vi "RunDelay2.vi"() -> ()   [LabVIEW 2009]
uses:
  BME Beispiele/BME DLL/DelayGenerator.dll
panel:
  out "error out":errorcluster
  in  "DEACTIVATE":bool
  out "output param 21":i32
  out "output param 13":i32
  out "output param 18":i32
  out "output param 7":u32
  out "output param 6":u32
  out "output param 17":i32
  out "output param 12":i32
  out "output param 11":i32
  in  "Internal Trigger":bool=TRUE
  in  "Trigger Period":dbl=10000.0
  out "output param 9":i32
  out "output param 8":i32
  in  "stop":bool
  in  "T(S) Delay":dbl
  in  "T(S) Reset":dbl
  in  "T(S) Active":bool=TRUE
  in  "A(S) Delay":dbl
  in  "A(S) Reset":dbl
  in  "A(S) Acitve":bool=TRUE
  in  "B(S) Delay":dbl=1000.0
  in  "B(S) Reset":dbl=4000.0
  in  "B(S) Acitve":bool=TRUE
  out "output param 14":u32
  out "output param 15":u32
  out "output param 16":u32
  out "output param 10":i32
  in  "T0 Active":bool=TRUE
  in  "T0 Delay":dbl
  in  "A  Delay":dbl
  in  "A  Active":bool=TRUE
  in  "B  Delay":dbl=1000.0
  in  "B  Active":bool=TRUE
  in  "Gate AB":bool=TRUE
  in  "Apply":bool
  out "output param 20":u32
  out "output param 19":u32
  out "output param 4":i32
  out "output param 5":i32
  out "output param 2":i32
  out "DG_ProductM":i32
  out "SlotNumberM":i32
  out "IsMaster?m":i32
  out "output param 3":i32
  out "DG_ProductS":i32
  out "SlotNumberS":i32
  out "IsMaster?s":i32
  out "DG_NumberM":i32
  out "DG_NumberS":i32
  out "output param 1":i32
  out "NumberOfCards Detected":i32
  out "p_Error 2":i32
  # "Info-Master"
  # "Info-Slave1"
  # "All error indicators are hidden.\nIn order to see a return value \nof some function, make the \nindicator visible (show indicator)"
  # "ALL TIME VALUES IN msek !"
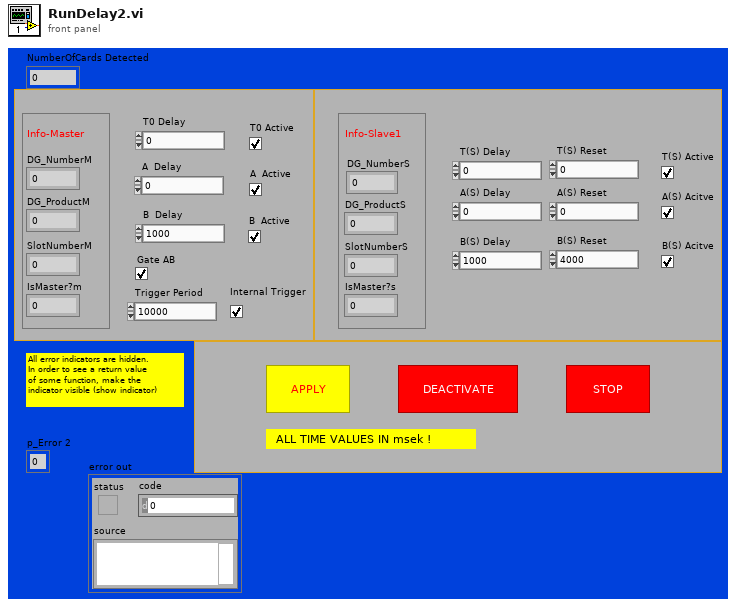
[diagram p1: front panel]
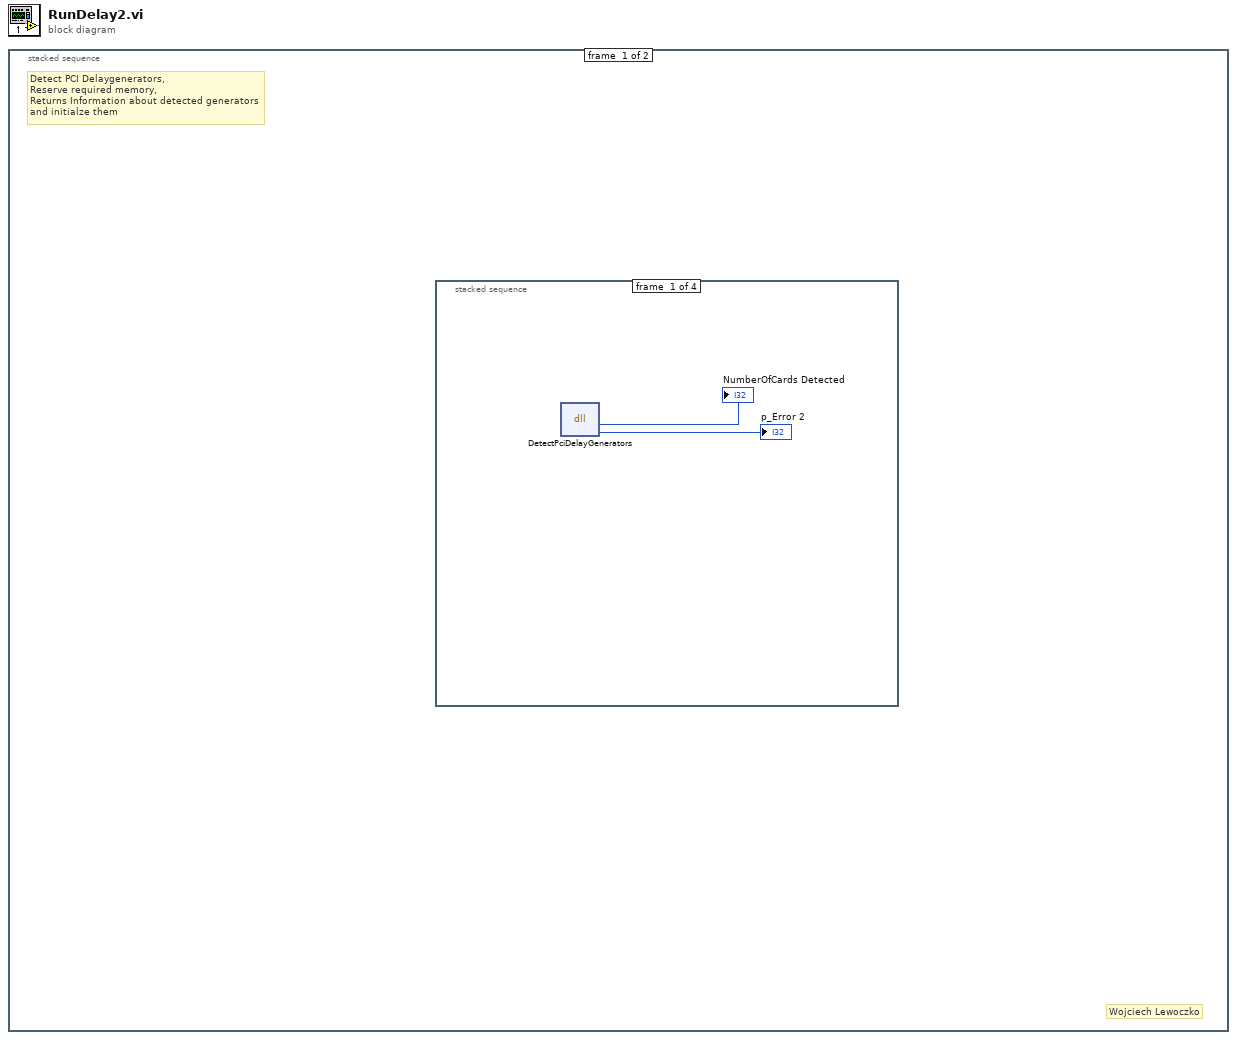
[diagram p0: block diagram]
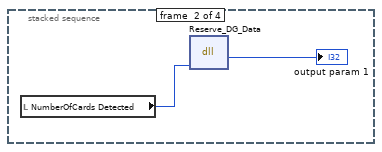
[diagram p2: hidden frame]
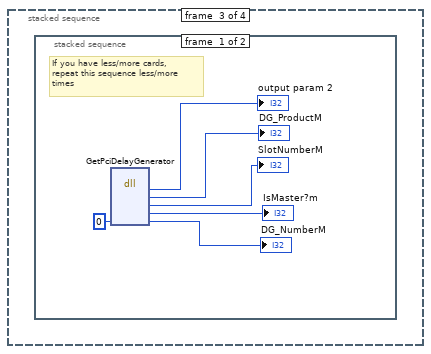
[diagram p3: hidden frame]
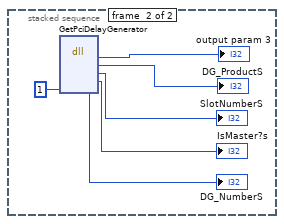
[diagram p4: hidden frame]
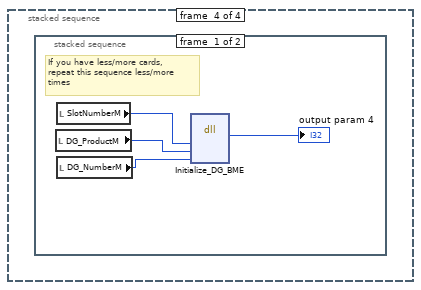
[diagram p5: hidden frame]
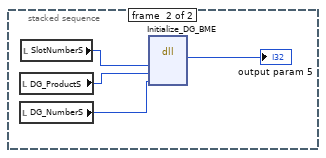
[diagram p6: hidden frame]
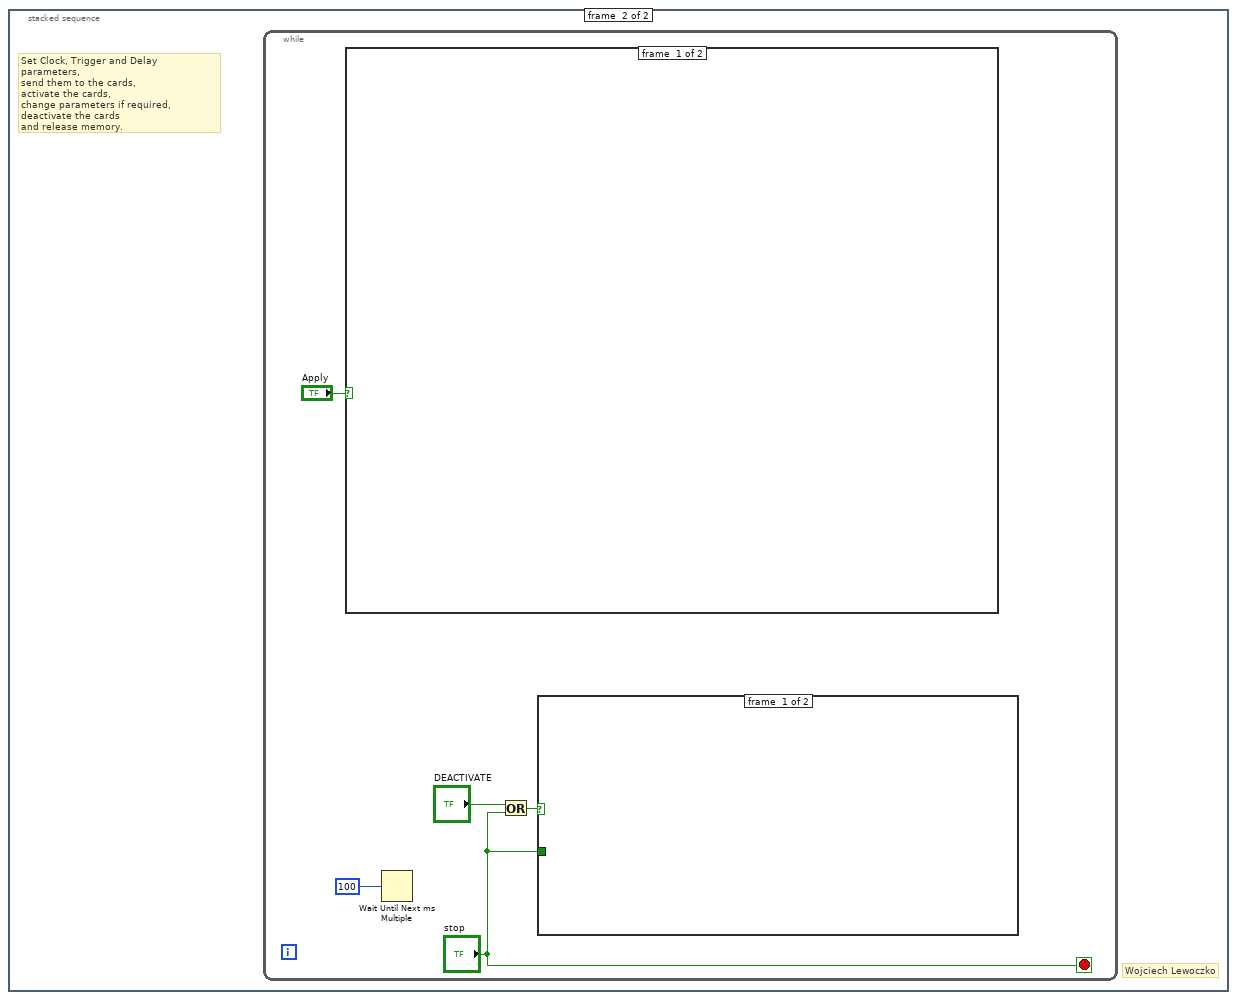
[diagram p7: hidden frame]
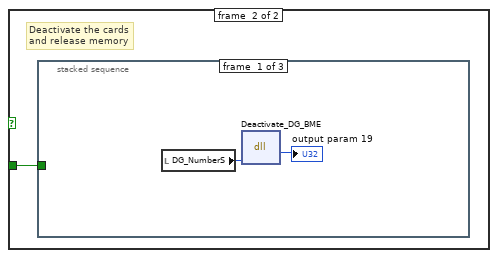
[diagram p8: hidden frame]
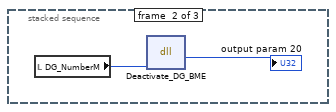
[diagram p9: hidden frame]
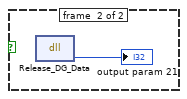
[diagram p11: hidden frame]
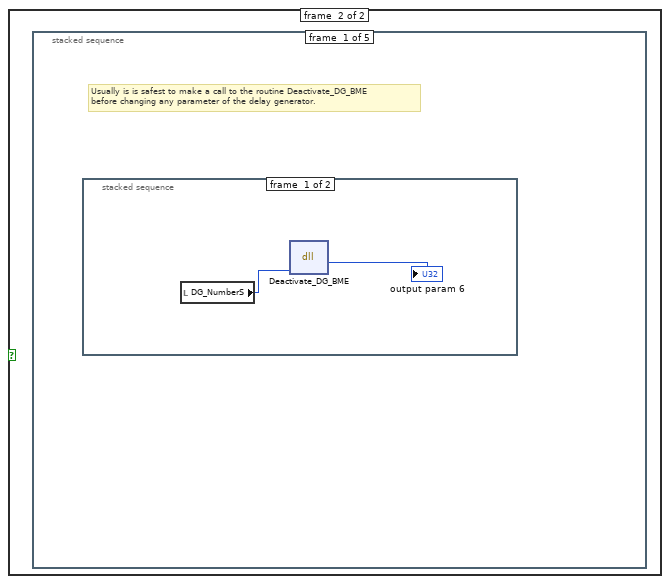
[diagram p12: hidden frame]
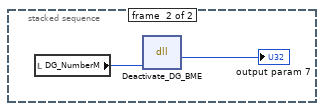
[diagram p13: hidden frame]
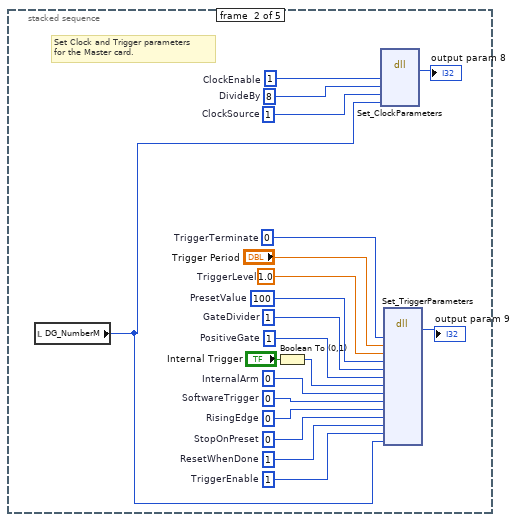
[diagram p14: hidden frame]
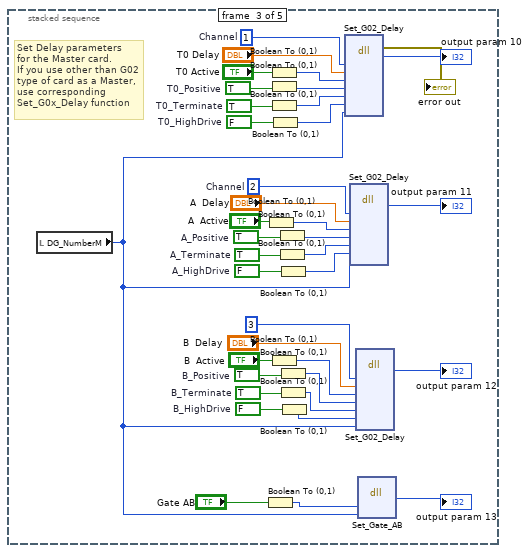
[diagram p15: hidden frame]
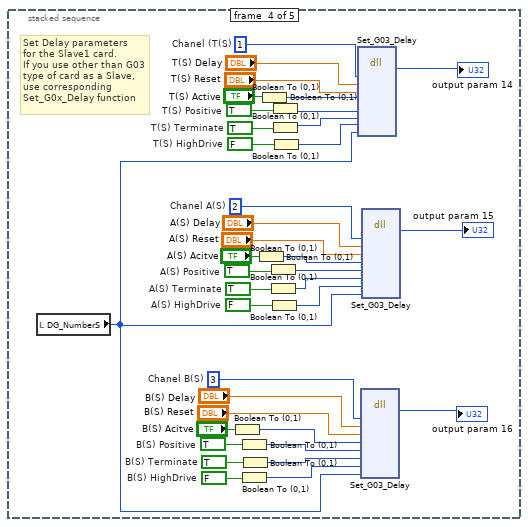
[diagram p16: hidden frame]
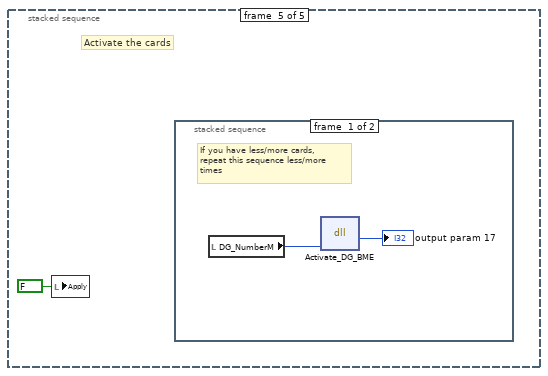
[diagram p17: hidden frame]
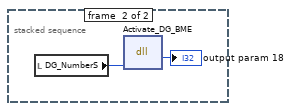
[diagram p18: hidden frame]
diagram:
  n1 = stacked-sequence {
    frame #0 {
      # "Wojciech Lewoczko"
      # "Detect PCI Delaygenerators,\nReserve required memory,\nReturns Information about detected generators \nand initialze them"
      n2 = stacked-sequence {
        frame #0 {
          n3 = dll-call lib="C:/Dokumente und Einstellungen/A2.5/Desktop/BME Beispiele/BME DLL/DelayGenerator.dll" fn="DetectPciDelayGenerators"() -> ("NumberOfCards"=→"NumberOfCards Detected":i32, "p_Error"=→"p_Error 2":i32)  [unwired: 4 in, 2 out]
        }
        frame #1 {
          n4 = local read "NumberOfCards Detected"() -> (w3:i32)
          n5 = dll-call lib="C:/Dokumente und Einstellungen/A2.5/Desktop/BME Beispiele/BME DLL/DelayGenerator.dll" fn="Reserve_DG_Data"("Number of cards"=w3) -> (→"output param 1":i32)  [unwired: 4 in, 2 out]
        }
        frame #2 {
          n6 = stacked-sequence {
            frame #0 {
              # "If you have less/more cards,\nrepeat this sequence less/more\ntimes"
              n7 = dll-call lib="C:/Dokumente und Einstellungen/A2.5/Desktop/BME Beispiele/BME DLL/DelayGenerator.dll" fn="GetPciDelayGenerator"("DG_Number"=0) -> (→"output param 2":i32, "DG_Product"=→"DG_ProductM":i32, "SlotNumber"=→"SlotNumberM":i32, "Master"=→"IsMaster?m":i32, "DG_Number"=→"DG_NumberM":i32)  [unwired: 6 in, 2 out]
            }
            frame #1 {
              n8 = dll-call lib="C:/Dokumente und Einstellungen/A2.5/Desktop/BME Beispiele/BME DLL/DelayGenerator.dll" fn="GetPciDelayGenerator"("DG_Number"=1) -> (→"output param 3":i32, "DG_Product"=→"DG_ProductS":i32, "SlotNumber"=→"SlotNumberS":i32, "Master"=→"IsMaster?s":i32, "DG_Number"=→"DG_NumberS":i32)  [unwired: 6 in, 2 out]
            }
          }
        }
        frame #3 {
          n9 = stacked-sequence {
            frame #0 {
              # "If you have less/more cards,\nrepeat this sequence less/more\ntimes"
              n10 = local read "DG_ProductM"() -> (w19:i32)
              n11 = local read "SlotNumberM"() -> (w18:i32)
              n12 = local read "DG_NumberM"() -> (w20:i32)
              n13 = dll-call lib="C:/Dokumente und Einstellungen/A2.5/Desktop/BME Beispiele/BME DLL/DelayGenerator.dll" fn="Initialize_DG_BME"("base"=w18, "Product"=w19, "DG_Number"=w20) -> (→"output param 4":i32)  [unwired: 6 in, 2 out]
            }
            frame #1 {
              n14 = local read "DG_ProductS"() -> (w22:i32)
              n15 = local read "DG_NumberS"() -> (w23:i32)
              n16 = local read "SlotNumberS"() -> (w21:i32)
              n17 = dll-call lib="C:/Dokumente und Einstellungen/A2.5/Desktop/BME Beispiele/BME DLL/DelayGenerator.dll" fn="Initialize_DG_BME"("base"=w21, "Product"=w22, "DG_Number"=w23) -> (→"output param 5":i32)  [unwired: 6 in, 2 out]
            }
          }
        }
      }
    }
    frame #1 {
      # "Wojciech Lewoczko"
      # "Set Clock, Trigger and Delay parameters,\nsend them to the cards,\nactivate the cards,\nchange parameters if required,\ndeactivate the cards\nand release memory."
      n18 = while {
        stop <- "stop" stop-if-true
        n19 = case shown="True" "Apply" {
          frame #0 {
          }
          frame #1 {
            n20 = stacked-sequence {
              frame #0 {
                # "Usually is is safest to make a call to the routine Deactivate_DG_BME \nbefore changing any parameter of the delay generator."
                n21 = stacked-sequence {
                  frame #0 {
                    n22 = local read "DG_NumberS"() -> (w37:i32)
                    n23 = dll-call lib="C:/Dokumente und Einstellungen/A2.5/Desktop/BME Beispiele/BME DLL/DelayGenerator.dll" fn="Deactivate_DG_BME"("DG_Number"=w37) -> (→"output param 6":u32)  [unwired: 4 in, 2 out]
                  }
                  frame #1 {
                    n24 = local read "DG_NumberM"() -> (w39:i32)
                    n25 = dll-call lib="C:/Dokumente und Einstellungen/A2.5/Desktop/BME Beispiele/BME DLL/DelayGenerator.dll" fn="Deactivate_DG_BME"("DG_Number"=w39) -> (→"output param 7":u32)  [unwired: 4 in, 2 out]
                  }
                }
              }
              frame #1 {
                w51 = 1.0  # TriggerLevel
                w41 = 1  # TriggerEnable
                w42 = 1  # ResetWhenDone
                w43 = 0  # StopOnPreset
                w44 = 0  # RisingEdge
                w45 = 0  # SoftwareTrigger
                w46 = 0  # InternalArm
                w48 = 1  # PositiveGate
                w49 = u32 1  # GateDivider
                w50 = u32 100  # PresetValue
                w53 = 0  # TriggerTerminate
                w58 = 1  # ClockSource
                w59 = u32 8  # DivideBy
                w60 = 1  # ClockEnable
                # "Set Clock and Trigger parameters\nfor the Master card."
                n26 = local read "DG_NumberM"() -> (w57:i32)
                n27 = Boolean To (0,1)(Boolean="Internal Trigger") -> (0, 1=w47:i16)
                n28 = dll-call lib="C:/Dokumente und Einstellungen/A2.5/Desktop/BME Beispiele/BME DLL/DelayGenerator.dll" fn="Set_ClockParameters"("ClockEnable"=w60, "DivideBy"=w59, "ClockSource"=w58, "DG_Number"=w57) -> (→"output param 8":i32)  [unwired: 7 in, 2 out]
                n29 = dll-call lib="C:/Dokumente und Einstellungen/A2.5/Desktop/BME Beispiele/BME DLL/DelayGenerator.dll" fn="Set_TriggerParameters"("TriggerTerminate"=w53, "InternalClock"="Trigger Period", "TriggerLevel"=w51, "PresetValue"=w50, "GateDivider"=w49, "PositiveGate"=w48, "InternalTrigger"=w47, "InternalArm"=w46, "SoftwareTrigger"=w45, "RisingEdge"=w44, "StopOnPreset"=w43, "ResetWhenDone"=w42, "TriggerEnable"=w41, "DG_Number"=w57) -> (→"output param 9":i32)  [unwired: 17 in, 2 out]
              }
              frame #2 {
                w77 = u32 2  # Channel
                w84 = u32 1  # Channel
                w85 = FALSE  # B_HighDrive
                w86 = TRUE  # B_Terminate
                w87 = TRUE  # B_Positive
                w88 = FALSE  # A_HighDrive
                w89 = TRUE  # A_Terminate
                w90 = TRUE  # A_Positive
                w91 = FALSE  # T0_HighDrive
                w92 = TRUE  # T0_Terminate
                w93 = TRUE  # T0_Positive
                # "Set Delay parameters\nfor the Master card.\nIf you use other than G02\ntype of card as a Master,\nuse corresponding \nSet_G0x_Delay function"
                n30 = local read "DG_NumberM"() -> (w63:i32)
                n31 = Boolean To (0,1)(Boolean="Gate AB") -> (0, 1=w64:i16)
                n32 = Boolean To (0,1)(Boolean="A  Active") -> (0, 1=w75:i16)
                n33 = Boolean To (0,1)(Boolean="T0 Active") -> (0, 1=w82:i16)
                n34 = Boolean To (0,1)(Boolean=w93) -> (0, 1=w81:i16)
                n35 = Boolean To (0,1)(Boolean=w92) -> (0, 1=w80:i16)
                n36 = Boolean To (0,1)(Boolean="B  Active") -> (0, 1=w68:i16)
                n37 = Boolean To (0,1)(Boolean=w91) -> (0, 1=w79:i16)
                n38 = Boolean To (0,1)(Boolean=w90) -> (0, 1=w74:i16)
                n39 = Boolean To (0,1)(Boolean=w89) -> (0, 1=w73:i16)
                n40 = Boolean To (0,1)(Boolean=w88) -> (0, 1=w72:i16)
                n41 = Boolean To (0,1)(Boolean=w87) -> (0, 1=w67:i16)
                n42 = Boolean To (0,1)(Boolean=w86) -> (0, 1=w66:i16)
                n43 = Boolean To (0,1)(Boolean=w85) -> (0, 1=w65:i16)
                n44 = dll-call lib="C:/Dokumente und Einstellungen/A2.5/Desktop/BME Beispiele/BME DLL/DelayGenerator.dll" fn="Set_G02_Delay"("Channel"=w84, "FireFirst"="T0 Delay", "Active"=w82, "Positive"=w81, "Terminate"=w80, "HighDrive"=w79, "DG_Number"=w63) -> (error out=→"error out":errorcluster, "Error"=→"output param 10":i32)  [unwired: 10 in, 1 out]
                n45 = dll-call lib="C:/Dokumente und Einstellungen/A2.5/Desktop/BME Beispiele/BME DLL/DelayGenerator.dll" fn="Set_G02_Delay"("Channel"=w77, "FireFirst"="A  Delay", "Active"=w75, "Positive"=w74, "Terminate"=w73, "HighDrive"=w72, "DG_Number"=w63) -> ("Error"=→"output param 11":i32)  [unwired: 10 in, 2 out]
                n46 = dll-call lib="C:/Dokumente und Einstellungen/A2.5/Desktop/BME Beispiele/BME DLL/DelayGenerator.dll" fn="Set_G02_Delay"("Channel"=u32 3, "FireFirst"="B  Delay", "Active"=w68, "Positive"=w67, "Terminate"=w66, "HighDrive"=w65, "DG_Number"=w63) -> ("Error"=→"output param 12":i32)  [unwired: 10 in, 2 out]
                n47 = dll-call lib="C:/Dokumente und Einstellungen/A2.5/Desktop/BME Beispiele/BME DLL/DelayGenerator.dll" fn="Set_Gate_AB"("Gate_AB"=w64, "DG_Number"=w63) -> (→"output param 13":i32)  [unwired: 5 in, 2 out]
              }
              frame #3 {
                w102 = FALSE  # B(S) HighDrive
                w103 = TRUE  # B(S) Terminate
                w104 = TRUE  # B(S) Positive
                w108 = FALSE  # A(S) HighDrive
                w109 = TRUE  # A(S) Terminate
                w110 = TRUE  # A(S) Positive
                w114 = FALSE  # T(S) HighDrive
                w115 = TRUE  # T(S) Terminate
                w116 = TRUE  # T(S) Positive
                w130 = u32 3  # Chanel B(S)
                w131 = u32 2  # Chanel A(S)
                w132 = u32 1  # Chanel (T(S)
                # "Set Delay parameters\nfor the Slave1 card.\nIf you use other than G03\ntype of card as a Slave,\nuse corresponding \nSet_G0x_Delay function"
                n48 = local read "DG_NumberS"() -> (w118:i32)
                n49 = Boolean To (0,1)(Boolean="B(S) Acitve") -> (0, 1=w122:i16)
                n50 = Boolean To (0,1)(Boolean=w104) -> (0, 1=w101:i16)
                n51 = Boolean To (0,1)(Boolean=w102) -> (0, 1=w99:i16)
                n52 = Boolean To (0,1)(Boolean=w103) -> (0, 1=w100:i16)
                n53 = Boolean To (0,1)(Boolean="A(S) Acitve") -> (0, 1=w125:i16)
                n54 = Boolean To (0,1)(Boolean="T(S) Active") -> (0, 1=w127:i16)
                n55 = Boolean To (0,1)(Boolean=w110) -> (0, 1=w107:i16)
                n56 = Boolean To (0,1)(Boolean=w109) -> (0, 1=w106:i16)
                n57 = Boolean To (0,1)(Boolean=w108) -> (0, 1=w105:i16)
                n58 = Boolean To (0,1)(Boolean=w116) -> (0, 1=w113:i16)
                n59 = Boolean To (0,1)(Boolean=w115) -> (0, 1=w112:i16)
                n60 = Boolean To (0,1)(Boolean=w114) -> (0, 1=w111:i16)
                n61 = dll-call lib="C:/Dokumente und Einstellungen/A2.5/Desktop/BME Beispiele/BME DLL/DelayGenerator.dll" fn="Set_G03_Delay"("Chanel"=w132, "FireFirst"="T(S) Delay", "Reset"="T(S) Reset", "Active"=w127, "Positive"=w113, "Terminate"=w112, "HighDrive"=w111, "DG_Number"=w118) -> (→"output param 14":u32)  [unwired: 11 in, 2 out]
                n62 = dll-call lib="C:/Dokumente und Einstellungen/A2.5/Desktop/BME Beispiele/BME DLL/DelayGenerator.dll" fn="Set_G03_Delay"("Chanel"=w130, "FireFirst"="B(S) Delay", "Reset"="B(S) Reset", "Active"=w122, "Positive"=w101, "Terminate"=w100, "HighDrive"=w99, "DG_Number"=w118) -> (→"output param 16":u32)  [unwired: 11 in, 2 out]
                n63 = dll-call lib="C:/Dokumente und Einstellungen/A2.5/Desktop/BME Beispiele/BME DLL/DelayGenerator.dll" fn="Set_G03_Delay"("Chanel"=w131, "FireFirst"="A(S) Delay", "Reset"="A(S) Reset", "Active"=w125, "Positive"=w107, "Terminate"=w106, "HighDrive"=w105, "DG_Number"=w118) -> (→"output param 15":u32)  [unwired: 11 in, 2 out]
              }
              frame #4 {
                # "Activate the cards"
                n64 = local write "Apply"(FALSE ("Apply")) -> ()
                n65 = stacked-sequence {
                  frame #0 {
                    # "If you have less/more cards,\nrepeat this sequence less/more\ntimes"
                    n66 = local read "DG_NumberM"() -> (w138:i32)
                    n67 = dll-call lib="C:/Dokumente und Einstellungen/A2.5/Desktop/BME Beispiele/BME DLL/DelayGenerator.dll" fn="Activate_DG_BME"("DG_Number"=w138) -> (→"output param 17":i32)  [unwired: 4 in, 2 out]
                  }
                  frame #1 {
                    n68 = local read "DG_NumberS"() -> (w139:i32)
                    n69 = dll-call lib="C:/Dokumente und Einstellungen/A2.5/Desktop/BME Beispiele/BME DLL/DelayGenerator.dll" fn="Activate_DG_BME"("DG_Number"=w139) -> (→"output param 18":i32)  [unwired: 4 in, 2 out]
                  }
                }
              }
            }
          }
        }
        n70 = Wait Until Next ms Multiple(millisecond multiple=u32 100) -> ()  [unwired: 1 out]
        n71 = Or(x="DEACTIVATE", y="stop") -> (x .or. y?=w27:bool)
        n72 = case shown="True" w27 {
          tunnel: "stop" -> [_ w30]
          frame #0 {
          }
          frame #1 {
            # "Deactivate the cards \nand release memory"
            n73 = stacked-sequence {
              tunnel: w30 -> [_ _ w35]
              frame #0 {
                n74 = local read "DG_NumberS"() -> (w31:i32)
                n75 = dll-call lib="C:/Dokumente und Einstellungen/A2.5/Desktop/BME Beispiele/BME DLL/DelayGenerator.dll" fn="Deactivate_DG_BME"("DG_Number"=w31) -> (→"output param 19":u32)  [unwired: 4 in, 2 out]
              }
              frame #1 {
                n76 = local read "DG_NumberM"() -> (w33:i32)
                n77 = dll-call lib="C:/Dokumente und Einstellungen/A2.5/Desktop/BME Beispiele/BME DLL/DelayGenerator.dll" fn="Deactivate_DG_BME"("DG_Number"=w33) -> (→"output param 20":u32)  [unwired: 4 in, 2 out]
              }
              frame #2 {
                n78 = case shown="True" w35 {
                  frame #0 {
                  }
                  frame #1 {
                    n79 = dll-call lib="C:/Dokumente und Einstellungen/A2.5/Desktop/BME Beispiele/BME DLL/DelayGenerator.dll" fn="Release_DG_Data"() -> (→"output param 21":i32)  [unwired: 3 in, 2 out]
                  }
                }
              }
            }
          }
        }
      }
    }
  }
